vi "Boolean 1D To Symbol.vi"(8 "Off":i32, 10 "Boolean Array":bool[](array[boolean]), 11 "On":i32) -> (2 "Symbols":i32[](array[numeric]))   [LabVIEW 2022 SP3]
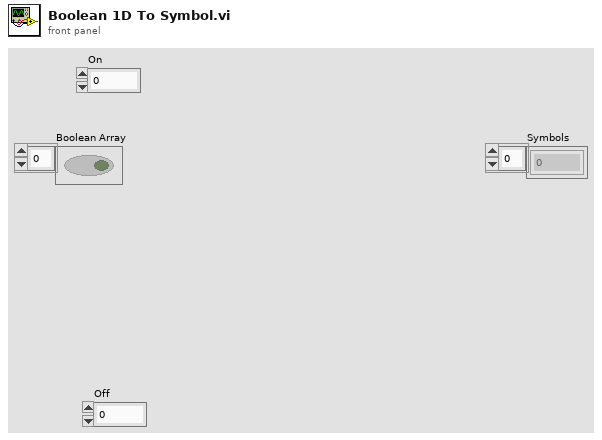
[diagram p1: front panel]
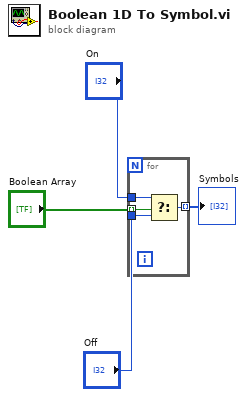
[diagram p0: block diagram]
diagram:
  n1 = for {
    tunnel: "Boolean Array" -> [w8] mode=indexing
    tunnel: "On" -> [w7]
    tunnel: "Off" -> [w6]
    tunnel: [w5] -> w1 mode=indexing
    n2 = Select(t=w7, s=w8, f=w6) -> (s? t:f=w5:i32)
  }
  "Symbols" <- w1
